vi "comprarcafe.vi"(8 "error in (no error)":errorcluster, 10 "Cluster":T1, 11 "UI Actor in":refnum<class "UI Actor.lvclass">) -> (0 "error out":errorcluster, 3 "UI Actor out":refnum<class "UI Actor.lvclass">)   [LabVIEW 2019, in "UI Actor.lvlib" / "UI Actor.lvclass"]
uses:
  UI Actor.lvclass
  C:/Program Files (x86)/National Instruments/LabVIEW 2019/vi.lib/ActorFramework/Actor/Actor.lvclass
  <vilib>/ActorFramework/Actor/Actor.lvclass/Actor.ctl
  <vilib>/ActorFramework/Message Enqueuer/Message Enqueuer.lvclass/Message Enqueuer.ctl
  UI Actor.lvclass/UI Actor.ctl
  <vilib>/ActorFramework/Message Enqueuer/Init from Existing Queue.vi
  <vilib>/ActorFramework/Message Enqueuer/Enqueue.vi
  UI Actor Messages/preciovscostocafe Msg/preciovscostocafe Msg.lvclass
  C:/Program Files (x86)/National Instruments/LabVIEW 2019/vi.lib/ActorFramework/Message/Message.lvclass
  <vilib>/ActorFramework/Message Priority Queue/Priority Enqueue.vi
  <vilib>/ActorFramework/Message Enqueuer/Message Enqueuer.lvclass
  <vilib>/ActorFramework/Actor/Actor.lvclass
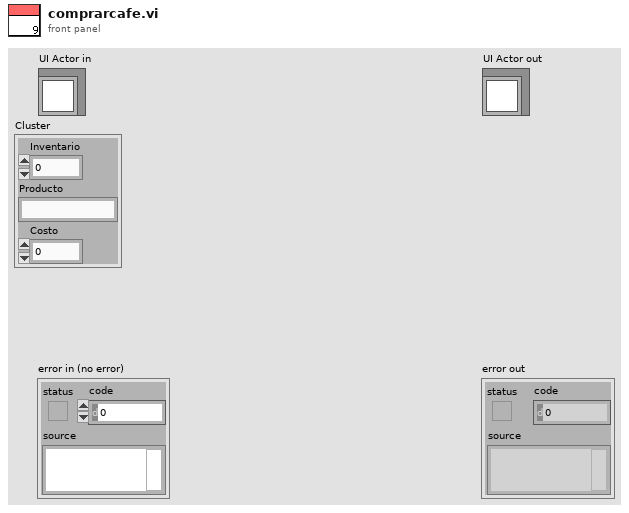
[diagram p1: front panel]
types:
  T1 = cluster{"Inventario":i32, "Producto":string, "Costo":dbl}
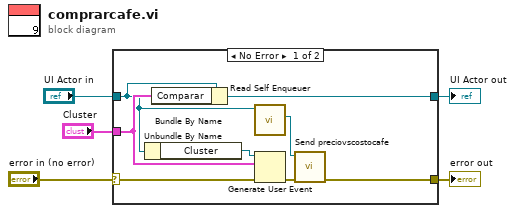
[diagram p0: block diagram]
diagram:
  n1 = case shown="No Error" "error in (no error)" {
    selector: "error in (no error)" -> [w12 w15]
    tunnel: [w7 w15] -> w4
    tunnel: [w11 w14] -> w2
    tunnel: "UI Actor in" -> [w9 w14]
    tunnel: "Cluster" -> [w10 _]
    frame No Error {
      n2 = Unbundle By Name(w9) -> ("Cluster"=w13:refnum<user-event>)
      n3 = Bundle By Name(cluster=w9, "Comparar"=w10) -> (w11:refnum<class "UI Actor.lvclass">)
      n4 = call <vilib>:"Read Self Enqueuer.vi"("Actor"=w9) -> ("Self Enqueuer"=w8:refnum<class "Message Enqueuer.lvclass">)  [unwired: 10 in]
      n5 = Generate User Event(user event=w13, event data cluster=w10, error in=w12) -> (error out=w6:errorcluster)  [unwired: 1 in, 1 out]
      n6 = call "Send preciovscostocafe.vi"("error in (no error)"=w6, "Message Enqueuer"=w8) -> ("error out"=w7:errorcluster)  [unwired: 8 in, 1 out]
    }
    frame Error {
    }
  }
  "error out" <- w4
  "UI Actor out" <- w2
